vi "Configure USB Compliance Test.vi"(6 "Adjacent Source (2: Ch 2)":u16(ring)=2 items=["Ch 1"=1, "Ch 2"=2, "Ch 3"=3, "Ch 4"=4], 7 "USB Test Type (0: Device Hi-Speed Signal Quality)":u16(ring) items=["Device Hi-Speed Signal Quality", "Host Hi-Speed Signal Quality", "Device Low Speed Signal Quality", "Host Low Speed Signal Quality", "Device Full Speed Signal Quality", "Host Full Speed Signal Quality"], 8 "error in (no error)":errorcluster, 9 "D- Probe Channel (3: Ch 3)":u16(ring)=3 items=["Ch 1"=1, "Ch 2"=2, "Ch 3"=3, "Ch 4"=4], 10 "D+ Probe Channel (1: Ch 1)":u16(ring)=1 items=["Ch 1"=1, "Ch 2"=2, "Ch 3"=3, "Ch 4"=4], 11 "VISA resource name":refnum<visa-resource-name>) -> (0 "error out":errorcluster, 3 "VISA resource name out":refnum<visa-resource-name>)   [LabVIEW 2015, in "Agilent 2000 3000 X-Series.lvlib"]
doc: "Configures the test type and sources for the test."
uses:
  <instrlib>/Agilent 2000 3000 X-Series/Agilent 2000 3000 X-Series.lvlib
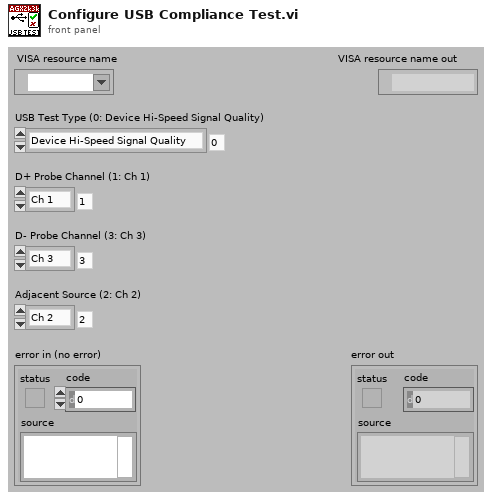
[diagram p1: front panel]
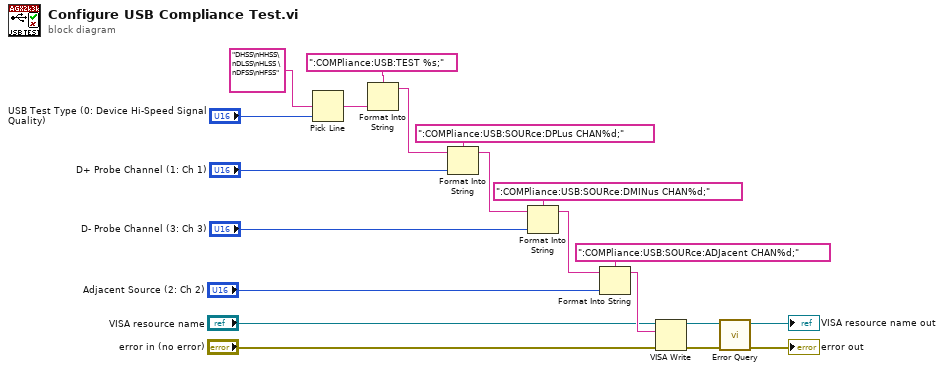
[diagram p0: block diagram]
diagram:
  n1 = Pick Line(multi-line string="DHSS\nHHSS\nDLSS\nHLSS \nDFSS\nHFSS", line index="USB Test Type (0: Device Hi-Speed Signal Quality)") -> (output string=w18:string)  [unwired: 1 in]
  n2 = Format Into String(format string=":COMPliance:USB:TEST %s;", w18) -> (resulting string=w16:string)  [unwired: 2 in, 1 out]
  n3 = Format Into String(format string=":COMPliance:USB:SOURce:DPLus CHAN%d;", initial string=w16, "D+ Probe Channel (1: Ch 1)") -> (resulting string=w12:string)  [unwired: 1 in, 1 out]
  n4 = Format Into String(format string=":COMPliance:USB:SOURce:DMINus CHAN%d;", initial string=w12, "D- Probe Channel (3: Ch 3)") -> (resulting string=w1:string)  [unwired: 1 in, 1 out]
  n5 = Format Into String(format string=":COMPliance:USB:SOURce:ADJacent CHAN%d;", initial string=w1, "Adjacent Source (2: Ch 2)") -> (resulting string=w8:string)  [unwired: 1 in, 1 out]
  n6 = VISA Write(VISA resource name="VISA resource name", write buffer=w8, error in (no error)="error in (no error)") -> (VISA resource name out=w7:refnum<visa-resource-name>, error out=w6:errorcluster)  [unwired: 1 out]
  n7 = call <instrlib>:"Error Query.vi"("error in (no error)"=w6, "VISA resource name"=w7) -> ("error out"=→"error out":errorcluster, "VISA resource name out"=→"VISA resource name out":refnum<visa-resource-name>)  [unwired: 6 in, 2 out]
